vi "例5.17  DDT数据类型转换成波形或数组.vi"() -> ()   [LabVIEW 2017]
panel:
  out "单一波形":waveform(dbl)
  out "数组":dbl[](array[numeric])
  out "单一波形":waveform(dbl) caption="单一波形1"
  out "波形数组":waveform(dbl)[](array[waveform])
  out "正弦":dynamicdata(graph) caption="仿真信号正弦"
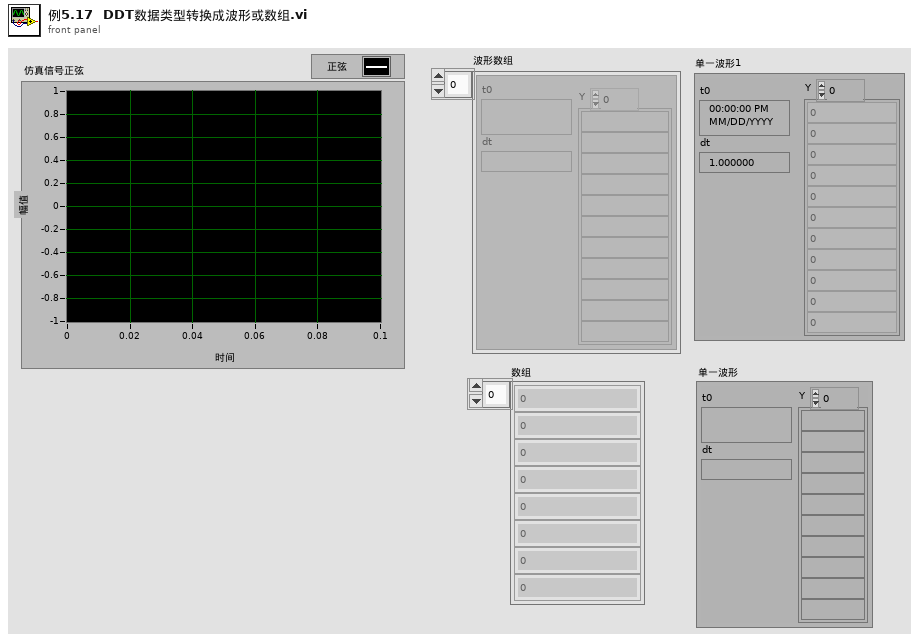
[diagram p1: front panel]
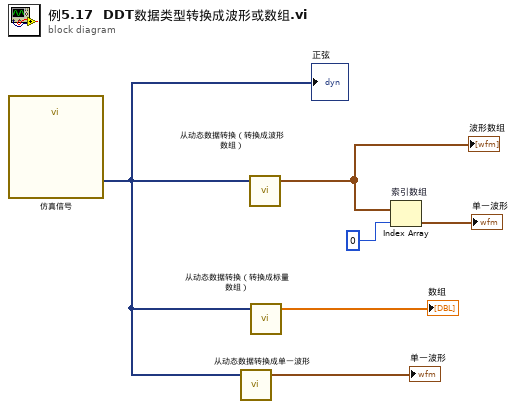
[diagram p0: block diagram]
diagram:
  n1 = call "仿真信号"() -> ("正弦"=w2:dynamicdata)  [unwired: 14 in, 1 out]
  "正弦" <- w2
  n2 = call "从动态数据转换成单一波形"("Dynamic Data Type"=w2) -> ("Waveform"=→"单一波形":waveform(dbl))  [unwired: 3 in]
  n3 = call "从动态数据转换（转换成波形数组）"("Dynamic Data Type"=w2) -> ("Array of Waveform"=w6:waveform(dbl)[])  [unwired: 3 in]
  "波形数组" <- w6
  n4 = call "从动态数据转换（转换成标量数组）"("Dynamic Data Type"=w2) -> ("Array"=→"数组":dbl[])  [unwired: 3 in]
  n5 = Index Array "索引数组"(array=w6, index=0 ("索引")) -> (element=→"单一波形":waveform(dbl))
